vi "Tools_KeyedArray Wildcard Index.vi"(4 "case matching (sensitive)":T1=enum."system", 5 "default value":string, 6 "wildcard key":string, 7 "array in":T2) -> (0 "match key":string, 1 "found key":bool, 2 "value":string, 3 "duplicate array":T2)   [LabVIEW 2012]
doc: "Returns the value of the first element whose key matches <B>wildcard key</B>."
uses:
  Tools_KeyedArray KeyedArray.ctl
  String/Tools_String Case Matching.ctl
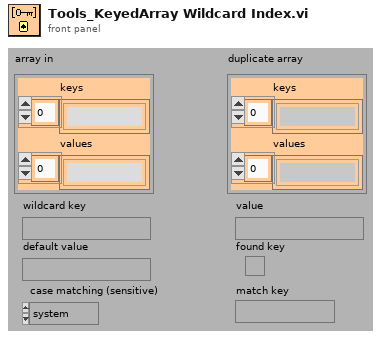
[diagram p1: front panel]
types:
  T1 = typedef "Tools_String Case Matching.ctl" = enum16{"a != A", "a == A", "system"}
  T2 = typedef "Tools_KeyedArray KeyedArray.ctl" = cluster{"keys":string[], "values":string[]}
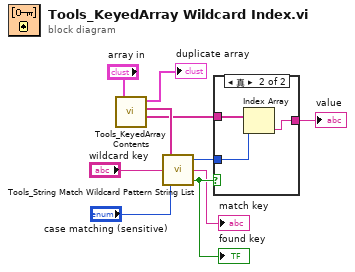
[diagram p0: block diagram]
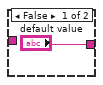
[diagram p2: hidden frame]
diagram:
  n1 = call "Tools_KeyedArray Contents.vi"("array in"="array in") -> ("values"=w6:string[], "keys"=w9:string[], "duplicate array"=→"duplicate array":T2)  [unwired: 4 out]
  n2 = call "Tools_String Match Wildcard Pattern String List.vi"("case matching (sensitive)"="case matching (sensitive)", "pattern"="wildcard key", "string list"=w9) -> ("found pattern"=w7:bool, "string"=→"match key":string, "index"=w3:i32)
  "found key" <- w7
  n3 = case shown="真" w7 {
    tunnel: w6 -> [_ w14]
    tunnel: ["default value" w13] -> w5
    tunnel: w3 -> [_ w12]
    frame False {
    }
    frame True {
      n4 = Index Array(array=w14, index=w12) -> (element=w13:string)
    }
  }
  "value" <- w5
